vi "MH_SetInputChannels.vi"(8 "error in (no error)":errorcluster caption="entrée d'erreur (pas d'erreur)", 10 "Channels new":T1[](array[typedef]) {"DeadTime" min=800 max=160000 step=1; "Edge" items=["falling", "rising"]; "Offset" min=-100000 max=100000 step=5; "Level" min=-1200 max=1200 step=1}, 11 "Channels old":T1[](array[typedef]) {"DeadTime" min=800 max=160000 step=1; "Edge" items=["falling", "rising"]; "Offset" min=-100000 max=100000 step=5; "Level" min=-1200 max=1200 step=1}) -> (0 "error out":errorcluster caption="sortie d'erreur", 2 "SetInpChan":T2[](array[typedef]), 3 "Channels":T1[](array[typedef]) {"DeadTime" min=800 max=160000 step=1; "Edge" items=["falling", "rising"]; "Offset" min=-100000 max=100000 step=5; "Level" min=-1200 max=1200 step=1})   [LabVIEW 2019]
uses:
  <userlib>/MultiHarp150/UIThread/MH_SetInpChanData.ctl
  <userlib>/MultiHarp150/UIThread/MH_SetInpChanCmds.ctl
  <userlib>/MultiHarp150/MH_InputChannel_LS.ctl
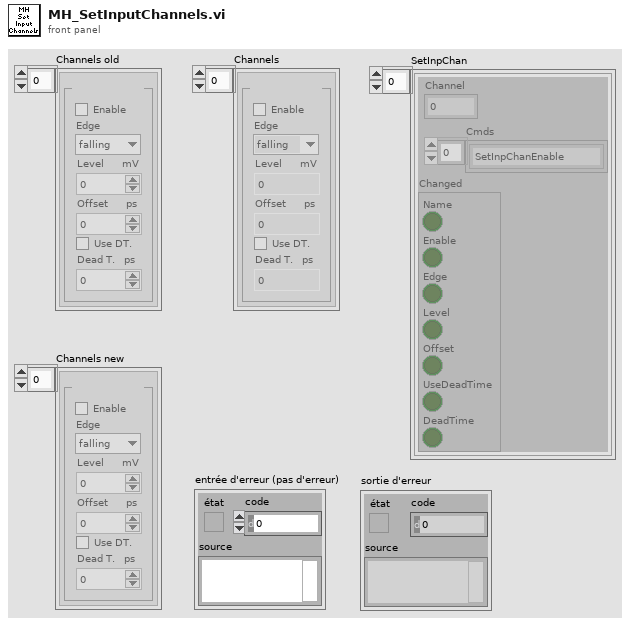
[diagram p1: front panel]
types:
  T1 = typedef "MH_InputChannel_LS.ctl" = cluster{"Name":string, "Enable":bool, "Edge":i32, "Level":i32, "Offset":i32, "UseDeadTime":bool, "DeadTime":i32}
  T2 = typedef "MH_SetInpChanData.ctl" = cluster{"Channel":i32, "Cmds":T3[], "Changed":cluster{"Name":bool, "Enable":bool, "Edge":bool, "Level":bool, "Offset":bool, "UseDeadTime":bool, "DeadTime":bool}}
  T3 = typedef "MH_SetInpChanCmds.ctl" = enum16{"SetInpChanEnable", "SetInpChanOffset", "SetInpChanDeadTime", "SetInpChanTrg"}
  T4 = cluster{"Name":bool, "Enable":bool, "Edge":bool, "Level":bool, "Offset":bool, "UseDeadTime":bool, "DeadTime":bool}[]
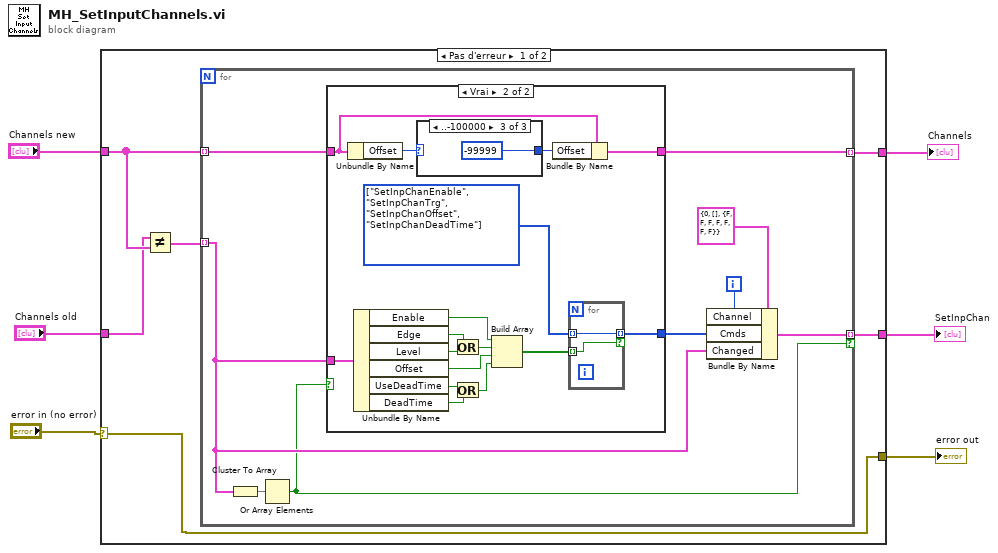
[diagram p0: block diagram]
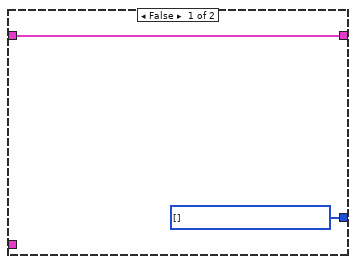
[diagram p2: hidden frame]
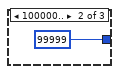
[diagram p4: hidden frame]
diagram:
  n1 = case shown="Pas d'erreur" "error in (no error)" {
    selector: "error in (no error)" -> [w8 w46]
    tunnel: [w12 w45] -> w6
    tunnel: "Channels new" -> [w11 w45]
    tunnel: "Channels old" -> [w9 _]
    tunnel: [w8 w46] -> w2
    tunnel: [w7 _] -> w1
    frame No Error {
      n2 = Not Equal?(x=w9, y=w11) -> (x != y?=w10:T4)
      n3 = for {
        tunnel: w10 -> [w16] mode=indexing
        tunnel: w11 -> [w20] mode=indexing
        tunnel: [w19] -> w12 mode=indexing
        tunnel: [w13] -> w7 mode=indexing if=w15
        i -> [w18]
        n4 = Cluster To Array(cluster=w16) -> (array=w21:bool[])
        n5 = Or Array Elements(Boolean array=w21) -> (logical OR=w15:bool)
        n6 = case shown="Vrai" w15 {
          tunnel: w16 -> [_ w39]
          tunnel: [w22 w24] -> w17
          tunnel: w20 -> [w23 w29]
          tunnel: [w23 w27] -> w19
          frame False {
            w22 = T3[] [] items=["SetInpChanEnable", "SetInpChanOffset", "SetInpChanDeadTime", "SetInpChanTrg"]
          }
          frame True {
            w26 = T3[] [enum."SetInpChanEnable", enum."SetInpChanTrg", enum."SetInpChanOffset", enum."SetInpChanDeadTime"] items=["SetInpChanEnable", "SetInpChanOffset", "SetInpChanDeadTime", "SetInpChanTrg"]
            n7 = Unbundle By Name(w29) -> ("Offset"=w30:i32)
            n8 = Unbundle By Name(w39) -> ("Enable"=w34:bool, "Edge"=w36:bool, "Level"=w35:bool, "Offset"=w32:bool, "UseDeadTime"=w37:bool, "DeadTime"=w38:bool)
            n9 = case shown="..-100000" w30 {
              selector: w30 -> [w42 _ _]
              tunnel: [w42 99999 ("SyncOffset") -99999 ("SyncOffset")] -> w28
              frame Default {
              }
              frame 100000.. {
              }
              frame ..-100000 {
              }
            }
            n10 = Or(x=w36, y=w35) -> (x .or. y?=w33:bool)
            n11 = Or(x=w37, y=w38) -> (x .or. y?=w31:bool)
            n12 = Build Array(w34, w33, w32, w31) -> (w25:bool[])
            n13 = Bundle By Name(cluster=w29, "Offset"=w28) -> (w27:T1)
            n14 = for {
              tunnel: w26 -> [w41] mode=indexing
              tunnel: w25 -> [w40] mode=indexing
              tunnel: [w41] -> w24 mode=indexing if=w40
            }
          }
        }
        n15 = Bundle By Name(cluster=T2 {"Channel"=0, "Cmds"=[], "Changed"={"Name"=FALSE, "Enable"=FALSE, "Edge"=FALSE, "Level"=FALSE, "Offset"=FALSE, "UseDeadTime"=FALSE, "DeadTime"=FALSE}} ("SetInpChanData"), "Channel"=w18, "Cmds"=w17, "Changed"=w16) -> (w13:T2)
      }
    }
    frame Error {
    }
  }
  "SetInpChan" <- w1
  "Channels" <- w6
  "error out" <- w2
